vi "Overlay arrows.vi"(8 "error in (no error)":errorcluster, 11 "OutputCluster":T1={"Acknowledgement"={"Enqueuer"=refnum, "VIReference"=refnum, "VIName"=""}, "AllPartInfo"=[{"PartName"="", "NumberOfRacks"=0, "MeasurementIDsArray"=[], "MeasurementNamesArray"=[], "SpecValuesArray"=[]}], "PartInfo"={"PartName"="", "TotalCount"=0, "ReelCount"=0, "NumberOfRacks"=0, "MeasurementIDsArray"=[], "MeasurementNamesArray"=[], "SpecValuesArray"=[]}, "Result Cluster"={"Measurement Names Array"=[], "Pass-Fail Array"=[], "Measurement Values Array "=[], "Roi for overlay (Arrows) Array"=[], "Algo Type Array"=[], "Image Array"=[], "Clamp operations"=enum."Average Clamp", "  Search Direction "=[], "Images_Array_in"=[], "ResultPF"=FALSE, "Total Cluster Values"={"Total Fail"=0, "Total Pass"=0, "Total Count"=0}, "Reel Counter Cluster"={"Reel Fail"=0, "Reel Pass"=0, "Reel Count"=0}, "Tolerance  Array"=[], "Array of Cam Spec Control Bool"=[], "Control Pass Fail Array"=[], "Specification Pass Fail Array"=[], "Overlay Arrow Lines"=[], "Camera ID"=[], "Trigger count"=0, "Specification fail?"=FALSE}, "ErrorMessage"=""}) -> (0 "error out":errorcluster)   [LabVIEW 2019, in "Algorithm.lvclass"]
uses:
  FrameworkOverrides/Algorithm.lvclass
  Common/Controls/AllPartInfo.ctl
  <vilib>/ActorFramework/Message Enqueuer/Message Enqueuer.lvclass
  Common/Controls/Acknowledgement.ctl
  Controls/Result Cluster.ctl
  Controls/OutputCluster.ctl
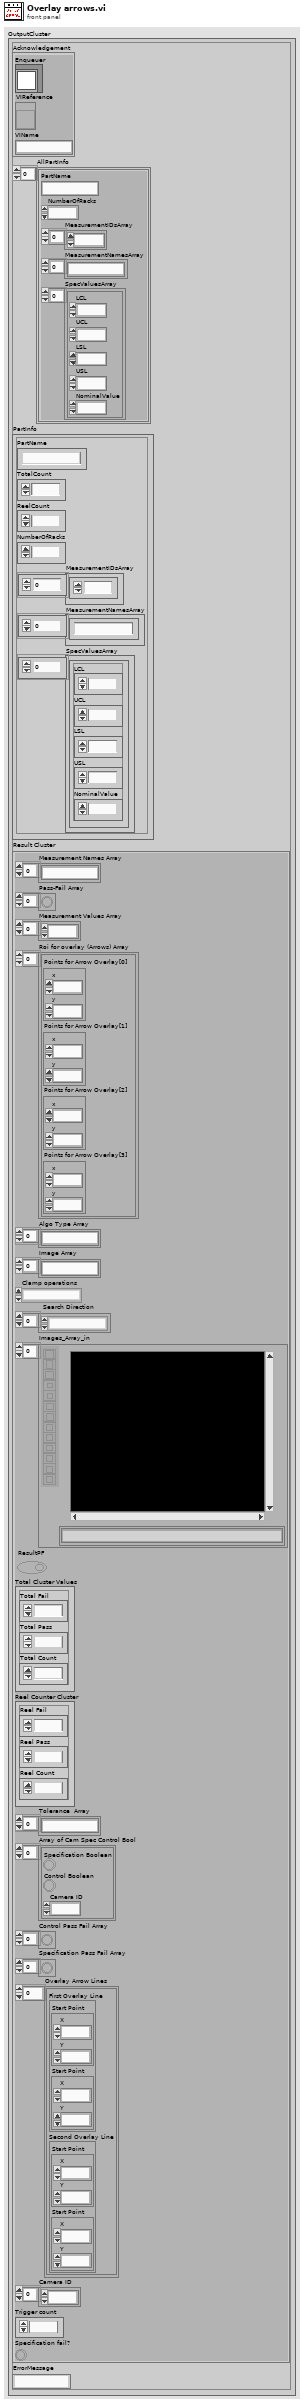
[diagram p1: front panel]
types:
  T1 = typedef "Algorithm.lvclass/OutputCluster.ctl" = cluster{"Acknowledgement":T2, "AllPartInfo":T3, "PartInfo":cluster{"PartName":string, "TotalCount":u64, "ReelCount":u64, "NumberOfRacks":u8, "MeasurementIDsArray":u16[], "MeasurementNamesArray":string[], "SpecValuesArray":cluster{"LCL":dbl, "UCL":dbl, "LSL":dbl, "USL":dbl, "NominalValue":dbl}[]}, "Result Cluster":T4, "ErrorMessage":string}
  T2 = typedef "Acknowledgement.ctl" = cluster{"Enqueuer":refnum<class "Message Enqueuer.lvclass">, "VIReference":refnum<vi>, "VIName":string}
  T3 = typedef "AllPartInfo.ctl" = cluster{"PartName":string, "NumberOfRacks":u8, "MeasurementIDsArray":u16[], "MeasurementNamesArray":string[], "SpecValuesArray":cluster{"LCL":dbl, "UCL":dbl, "LSL":dbl, "USL":dbl, "NominalValue":dbl}[]}[]
  T4 = typedef "Algorithm.lvclass/Result Cluster.ctl" = cluster{"Measurement Names Array":string[], "Pass-Fail Array":bool[], "Measurement Values Array ":dbl[], "Roi for overlay (Arrows) Array":cluster{"Points for Arrow Overlay[0]":cluster{"x":dbl, "y":dbl}, "Points for Arrow Overlay[1]":cluster{"x":dbl, "y":dbl}, "Points for Arrow Overlay[2]":cluster{"x":dbl, "y":dbl}, "Points for Arrow Overlay[3]":cluster{"x":dbl, "y":dbl}}[], "Algo Type Array":string[], "Image Array":string[], "Clamp operations":enum16{"Min Clamp", "Max Clamp", "Average Clamp"}, "  Search Direction ":enum16{"Left to Right", "Right to Left", "Top to Bottom", "Bottom to Top"}[], "Images_Array_in":T5[], "ResultPF":bool, "Total Cluster Values":cluster{"Total Fail":u64, "Total Pass":u64, "Total Count":u64}, "Reel Counter Cluster":cluster{"Reel Fail":u64, "Reel Pass":u64, "Reel Count":u64}, "Tolerance  Array":string[], "Array of Cam Spec Control Bool":cluster{"Specification Boolean":bool, "Control Boolean":bool, "Camera ID":i8}[], "Control Pass Fail Array":bool[], "Specification Pass Fail Array":bool[], "Overlay Arrow Lines":cluster{"First Overlay Line ":cluster{"Start Point":cluster{"X":sgl, "Y":sgl}, "Start Point":cluster{"X":sgl, "Y":sgl}}, "Second Overlay Line ":cluster{"Start Point":cluster{"X":sgl, "Y":sgl}, "Start Point":cluster{"X":sgl, "Y":sgl}}}[], "Camera ID":i8[], "Trigger count":i32, "Specification fail?":bool}
  T5 = typedef "IMAQ Image.ctl" = refnum<image>
  T6 = cluster{"First Overlay Line ":cluster{"Start Point":cluster{"X":sgl, "Y":sgl}, "Start Point":cluster{"X":sgl, "Y":sgl}}, "Second Overlay Line ":cluster{"Start Point":cluster{"X":sgl, "Y":sgl}, "Start Point":cluster{"X":sgl, "Y":sgl}}}[]
  T7 = cluster{"Desired Font (Application)":enum16{"User-specified Font", "Application Font", "System Font", "Dialog Font"}, "[User-specified Font]":cluster{"Font Name":string, "Size":i16, "Strikeout?":bool, "Italic?":bool, "Underline?":bool, "Outline?":bool, "Shadow?":bool, "Bold?":bool, "Rotation Angle":dbl}, "Horizontal Alignment":i16, "Vertical Alignment":i16}
  T8 = cluster{"Start Point":cluster{"X":sgl, "Y":sgl}, "Start Point":cluster{"X":sgl, "Y":sgl}}
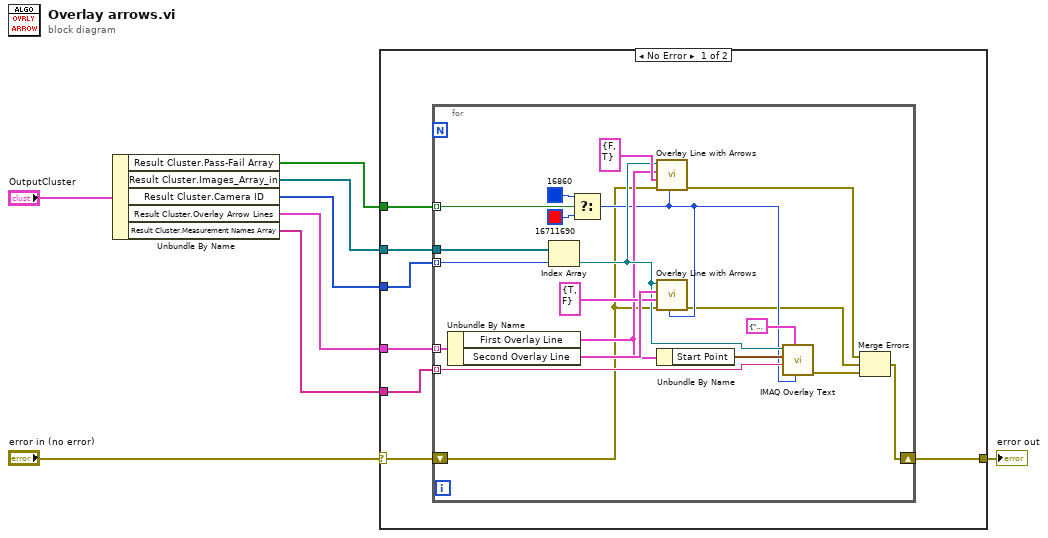
[diagram p0: block diagram]
diagram:
  n1 = Unbundle By Name("OutputCluster") -> ("Result Cluster.Pass-Fail Array"=w5:bool[], "Result Cluster.Images_Array_in"=w4:T5[], "Result Cluster.Camera ID"=w3:i8[], "Result Cluster.Overlay Arrow Lines"=w2:T6, "Result Cluster.Measurement Names Array"=w1:string[])
  n2 = case shown="No Error" "error in (no error)" {
    selector: "error in (no error)" -> [w10 w36]
    tunnel: w5 -> [w15 _]
    tunnel: w4 -> [w14 _]
    tunnel: w3 -> [w13 _]
    tunnel: w2 -> [w12 _]
    tunnel: w1 -> [w11 _]
    tunnel: [w9 w36] -> w7
    frame No Error {
      n3 = for {
        tunnel: w12 -> [w34] mode=indexing
        tunnel: w13 -> [w35] mode=indexing
        tunnel: w14 -> [w33]
        tunnel: w15 -> [w24] mode=indexing
        tunnel: w11 -> [w26] mode=indexing
        shift-right: [w16] -> w9
        shift-left: w10 -> [w20]
        n4 = Unbundle By Name(w34) -> ("First Overlay Line"=w28:T8, "Second Overlay Line"=w32:T8)
        n5 = Index Array(array=w33, index=w35) -> (element=w29:T5)
        n6 = Select(t=u32 16860 ("Color"), s=w24, f=u32 16711690 ("Color")) -> (s? t:f=w21:u32)
        n7 = call <vilib>:"Overlay Line with Arrows.vi"("Color"=w21, "error in (no error)"=w20, "Arrows"=cluster{"Start point":bool, "End point":bool} {"Start point"=FALSE, "End point"=TRUE}, "Line Coordinates"=w28, "Image In"=w29) -> ("error out"=w19:errorcluster)  [unwired: 5 in, 1 out]
        n8 = call <vilib>:"Overlay Line with Arrows.vi"("Color"=w21, "error in (no error)"=w20, "Arrows"=cluster{"Start point":bool, "End point":bool} {"Start point"=TRUE, "End point"=FALSE}, "Line Coordinates"=w32, "Image In"=w29) -> ("error out"=w18:errorcluster)  [unwired: 5 in, 1 out]
        n9 = Unbundle By Name(w28) -> ("Start Point"=w27:cluster{"X":sgl, "Y":sgl})
        n10 = call "IMAQ Overlay Text"("Text Color (black)"=w21, "Font, Size & Style"=T7 {"Desired Font (Application)"=enum."Application Font", "[User-specified Font]"={"Font Name"="Arial", "Size"=20, "Strikeout?"=FALSE, "Italic?"=FALSE, "Underline?"=FALSE, "Outline?"=FALSE, "Shadow?"=FALSE, "Bold?"=TRUE, "Rotation Angle"=0.0}, "Horizontal Alignment"=0, "Vertical Alignment"=0}, "String"=w26, "Origin"=w27, "Image"=w29) -> ("error out"=w17:errorcluster)  [unwired: 5 in, 1 out]
        n11 = Merge Errors(w19, w18, w17) -> (w16:errorcluster)
      }
    }
    frame Error {
    }
  }
  "error out" <- w7
